vi "Address Space Size.vi"(2 "AO in":refnum<class "Analog Output.lvclass">) -> (6 "size":u32)   [LabVIEW 2017, in "Analog IO.lvlib" / "Analog Output.lvclass"]
uses:
  Analog Output.lvclass
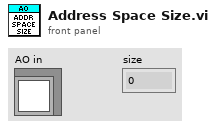
[diagram p1: front panel]
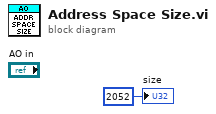
[diagram p0: block diagram]
diagram:
  "size" <- u32 2052 ("size")
